vi "GV_YscaleDrawScale.vi"(5 "[user-specified font]":T2, 6 "scale attributes":T1, 7 "desired font(Application)":T3(ring)=enum."Application Font", 8 "tick length(3)":i16=3, 9 "constant coordinate":i16=5, 10 "scale specs":cluster{"coordinate":i16, "label":string}[](array[cluster])=[{"coordinate"=7, "label"="1"}, {"coordinate"=23, "label"="2"}], 11 "picture":picture) -> (3 "new picture":picture)   [LabVIEW 2020, in "Sgraph_lib_V1.lvlib" / "Gviewer.lvclass"]
doc: "Andre Koelewijn, 25 July 2021\nDraw Y-scale on canvas"
uses:
  Gviewer.lvclass
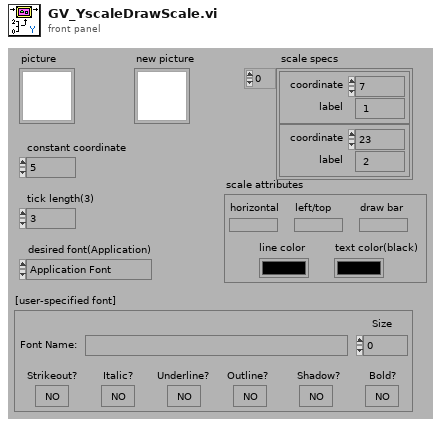
[diagram p1: front panel]
types:
  T1 = cluster{"horizontal":bool, "left/top":bool, "draw bar":bool, "line color":u32, "text color(black)":u32}
  T2 = cluster{"Font Name:":string, "Size":i16, "Strikeout?":bool, "Italic?":bool, "Underline?":bool, "Outline?":bool, "Shadow?":bool, "Bold?":bool}
  T3 = enum16{"User-specified Font", "Application Font", "System Font", "Dialog Font"}
  T4 = cluster{"constant coordinate":i16, "coordinate":i16}
  T5 = cluster{"coordinate":i16, "constant coordinate":i16}
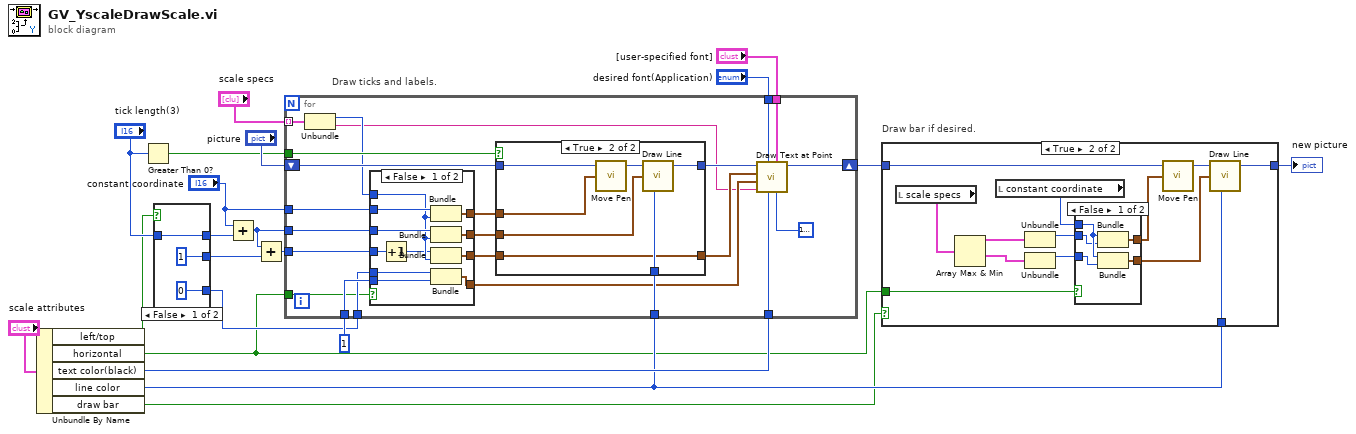
[diagram p0: block diagram]
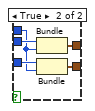
[diagram p3: hidden frame]
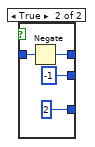
[diagram p4: hidden frame]
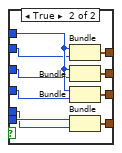
[diagram p5: hidden frame]
diagram:
  n1 = Unbundle By Name("scale attributes") -> ("left/top"=w5:bool, "horizontal"=w1:bool, "text color(black)"=w4:u32, "line color"=w3:u32, "draw bar"=w2:bool)
  n2 = Greater Than 0?(x="tick length(3)") -> (x > 0?=w16:bool)
  n3 = case shown="False" w5 {
    tunnel: "tick length(3)" -> [w24 w28]
    tunnel: [w24 w27] -> w12
    tunnel: [i16 1 i16 -1] -> w14
    tunnel: [0 2] -> w9
    frame False {
    }
    frame True {
      n4 = Negate(x=w28) -> (-x=w27:i16)
    }
  }
  n5 = Add(x="constant coordinate", y=w12) -> (x+y=w11:i16)
  n6 = Add(x=w11, y=w14) -> (x+y=w13:i16)
  n7 = for "Draw ticks and labels." {
    tunnel: "scale specs" -> [w51] mode=indexing
    tunnel: "constant coordinate" -> [w45]
    shift-right: [w34] -> w7
    shift-left: "picture" -> [w50]
    tunnel: "[user-specified font]" -> [w29]
    tunnel: "desired font(Application)" -> [w30]
    tunnel: w11 -> [w46]
    tunnel: w13 -> [w47]
    tunnel: w3 -> [w49]
    tunnel: w4 -> [w33]
    tunnel: w16 -> [w48]
    tunnel: 1 -> [w44]
    tunnel: w9 -> [w43]
    tunnel: w1 -> [w39]
    n8 = Unbundle(w51) -> ("coordinate"=w38:i16, "label"=w31:string)
    n9 = case shown="False" w39 {
      tunnel: w47 -> [w62 w65]
      tunnel: w46 -> [w61 w66]
      tunnel: w45 -> [w60 w67]
      tunnel: w38 -> [w59 w68]
      tunnel: w44 -> [w58 w64]
      tunnel: w43 -> [w57 w63]
      tunnel: [w56 w72] -> w37
      tunnel: [w55 w71] -> w42
      tunnel: [w54 w70] -> w41
      tunnel: [w53 w69] -> w40
      frame False {
        n10 = Increment(x=w62) -> (x+1=w52:i16)
        n11 = Bundle("constant coordinate"=w60, "coordinate"=w59) -> (w55:T4)  [unwired: 1 in]
        n12 = Bundle(w61, "coordinate"=w59) -> (w54:cluster{i16, "coordinate":i16})  [unwired: 1 in]
        n13 = Bundle(w52, "coordinate"=w59) -> (w53:cluster{i16, "coordinate":i16})  [unwired: 1 in]
        n14 = Bundle(w57, w58) -> (w56:cluster{i32, i32})  [unwired: 1 in]
      }
      frame True {
        n15 = Bundle("coordinate"=w68, "constant coordinate"=w67) -> (w71:T5)  [unwired: 1 in]
        n16 = Bundle("coordinate"=w68, w66) -> (w70:cluster{"coordinate":i16, i16})  [unwired: 1 in]
        n17 = Bundle("coordinate"=w68, w65) -> (w69:cluster{"coordinate":i16, i16})  [unwired: 1 in]
        n18 = Bundle(w64, w63) -> (w72:cluster{i32, i32})  [unwired: 1 in]
      }
    }
    n19 = case shown="True" w48 {
      tunnel: [w74 w80] -> w35
      tunnel: w50 -> [w74 w79]
      tunnel: w49 -> [_ w78]
      tunnel: w42 -> [w73 w77]
      tunnel: w41 -> [_ w76]
      tunnel: [w73 w75] -> w36
      tunnel: w40 -> [_ w75]
      frame False {
      }
      frame True {
        n20 = call <vilib>:"Move Pen.vi"("new position"=w77, "picture"=w79) -> ("new picture"=w81:picture)  [unwired: 3 in]
        n21 = call <vilib>:"Draw Line.vi"("picture"=w81, "end point"=w76, "color(black)"=w78) -> ("new picture"=w80:picture)  [unwired: 6 in]
      }
    }
    n22 = call <vilib>:"Draw Text at Point.vi"("BG color(transparent)"=u32 16777216, "[user-specified font]"=w29, "text color(black)"=w33, "desired font(Application)"=w30, "text"=w31, "alignment(left, top)"=w37, "origin"=w36, "picture"=w35) -> ("new picture"=w34:picture)  [unwired: 2 in, 1 out]
  }
  n23 = case "Draw bar if desired." shown="True" w2 {
    tunnel: [w82 w95] -> w8
    tunnel: w7 -> [w82 w93]
    tunnel: w3 -> [_ w92]
    tunnel: w1 -> [_ w89]
    frame False {
    }
    frame True {
      n24 = local read "scale specs"() -> (w87:cluster{"coordinate":i16, "label":string}[])
      n25 = Array Max & Min(array=w87) -> (max value=w85:cluster{"coordinate":i16, "label":string}, min value=w83:cluster{"coordinate":i16, "label":string})  [unwired: 2 out]
      n26 = local read "constant coordinate"() -> (w88:i16)
      n27 = Unbundle(w85) -> ("coordinate"=w86:i16)  [unwired: 1 out]
      n28 = Unbundle(w83) -> ("coordinate"=w84:i16)  [unwired: 1 out]
      n29 = case shown="False" w89 {
        tunnel: [w99 w105] -> w91
        tunnel: [w100 w104] -> w90
        tunnel: w88 -> [w98 w101]
        tunnel: w86 -> [w97 w103]
        tunnel: w84 -> [w96 w102]
        frame False {
          n30 = Bundle("constant coordinate"=w98, "coordinate"=w97) -> (w100:T4)  [unwired: 1 in]
          n31 = Bundle("constant coordinate"=w98, "coordinate"=w96) -> (w99:T4)  [unwired: 1 in]
        }
        frame True {
          n32 = Bundle("coordinate"=w103, "constant coordinate"=w101) -> (w104:T5)  [unwired: 1 in]
          n33 = Bundle("coordinate"=w102, "constant coordinate"=w101) -> (w105:T5)  [unwired: 1 in]
        }
      }
      n34 = call <vilib>:"Move Pen.vi"("new position"=w90, "picture"=w93) -> ("new picture"=w94:picture)  [unwired: 3 in]
      n35 = call <vilib>:"Draw Line.vi"("picture"=w94, "end point"=w91, "color(black)"=w92) -> ("new picture"=w95:picture)  [unwired: 6 in]
    }
  }
  "new picture" <- w8
